vi "G2CPU Treshold Detection.vi"(4 "Auto Release Treshold Parameters (Enabled)":T3={"Auto Release Treshold (Enabled)"=TRUE, "Auto Release Rising Edge (Enabled)"=TRUE}, 6 "Auto Release Line Profiles (Enabled)":T2={"Auto Release Line Profiles (Enabled)"=TRUE, "Auto Release Keys (Enabled)"=TRUE}, 8 "error in (no error)":errorcluster, 10 "Treshold Parameters":T1, 11 "Line Profiles":T4) -> (0 "error out":errorcluster, 3 "Edge Indexes out":refnum<class "1D Array f32.lvclass">)   [LabVIEW 2020, in "G2CPU Line Profile.lvlib"]
doc: "Find the location of the first treshold transition in each provided line profile.\nThe treshold parameters are executed on a per key basis.\nThe edge indexes put out are the indexes in the line profile where the treshold is found."
uses:
  G2CPU Line Profile.lvlib
  <vilib>/Natan Biesmans/G2CPU GPU and CPU HPC Toolkit/G2CPU Libraries/Arrays/1DArray/f32/1D Array f32.lvclass
  C:/Program Files/National Instruments/LabVIEW 2025/vi.lib/Natan Biesmans/G2CPU GPU and CPU HPC Toolkit/G2CPU Libraries/Arrays/Array/Array Prototype.lvclass
  <vilib>/Natan Biesmans/G2CPU GPU and CPU HPC Toolkit/G2CPU Libraries/Arrays/2DArray/f32/2D Array f32.lvclass
  <vilib>/Natan Biesmans/G2CPU GPU and CPU HPC Toolkit/G2CPU Libraries/Arrays/2DArray/u32/2D Array u32.lvclass
  <vilib>/Natan Biesmans/G2CPU GPU and CPU HPC Toolkit/G2CPU Libraries/Arrays/1DArray/binary/1D Array binary.lvclass
  <vilib>/Natan Biesmans/G2CPU GPU and CPU HPC Toolkit/G2CPU Libraries/Arrays/1DArray/s32/1D Array s32.lvclass
  <vilib>/Natan Biesmans/G2CPU GPU and CPU HPC Toolkit/G2CPU Libraries/Arrays/Array/Array Prototype.lvclass/Array Prototype.ctl
  d899a25e-58d2-4af9-a8d1-4a182ea10fc8.vi
  a0a0600d-4521-4ad1-868a-d08d3e0fc7ce.vi
  ee5f6664-b0a7-4185-b73b-108c1a354337.vi
  dc3a3043-0922-4d92-8bdc-4d35e29345f6.vi
  c8160532-a8a2-4c2d-9996-77c21ebed38b.vi
  7a05fecc-ed5d-4a87-a0b2-d0c328027071.vi
  <vilib>/Natan Biesmans/G2CPU GPU and CPU HPC Toolkit/G2CPU Libraries/Arrays/Array/G2CPU Get Array Pointer.vi
  d899a25e-58d2-4af9-a8d1-4a182ea10fc8.vi/2e03f477-51b7-4ba0-bb4f-4f838f6557e6.vi
  d899a25e-58d2-4af9-a8d1-4a182ea10fc8.vi/125d45d4-836b-469d-8a4a-6adb452f866d.vi
  d899a25e-58d2-4af9-a8d1-4a182ea10fc8.vi/8038e9ed-2e71-4568-91ba-0d873494c5ed.vi
  a0a0600d-4521-4ad1-868a-d08d3e0fc7ce.vi/2e03f477-51b7-4ba0-bb4f-4f838f6557e6.vi
  a0a0600d-4521-4ad1-868a-d08d3e0fc7ce.vi/125d45d4-836b-469d-8a4a-6adb452f866d.vi
  a0a0600d-4521-4ad1-868a-d08d3e0fc7ce.vi/8038e9ed-2e71-4568-91ba-0d873494c5ed.vi
  ee5f6664-b0a7-4185-b73b-108c1a354337.vi/cf27cc0d-1fb9-4e2f-ac40-7e8a0db6b27f.vi
  ee5f6664-b0a7-4185-b73b-108c1a354337.vi/1874d702-7e82-49f0-9e52-8a9dc00bddc1.vi
  ee5f6664-b0a7-4185-b73b-108c1a354337.vi/d603c635-5557-46f9-9702-9944444483a4.vi
  dc3a3043-0922-4d92-8bdc-4d35e29345f6.vi/a7ec311c-7cd8-4650-9526-d70ff0a769d1.vi
  c8160532-a8a2-4c2d-9996-77c21ebed38b.vi/5793b77b-c002-4ebf-9075-685617c95341.vi
  c8160532-a8a2-4c2d-9996-77c21ebed38b.vi/2ed3ef86-c00d-4d71-b84c-20267a6dfcf9.vi
  7a05fecc-ed5d-4a87-a0b2-d0c328027071.vi/d8e2d9cc-c923-495e-b121-b6b84788c73f.vi
  7a05fecc-ed5d-4a87-a0b2-d0c328027071.vi/345e91f0-9a5e-4de4-af9c-133346717e4a.vi
  d899a25e-58d2-4af9-a8d1-4a182ea10fc8.vi/2e03f477-51b7-4ba0-bb4f-4f838f6557e6.vi/d8e2d9cc-c923-495e-b121-b6b84788c73f.vi
  d899a25e-58d2-4af9-a8d1-4a182ea10fc8.vi/2e03f477-51b7-4ba0-bb4f-4f838f6557e6.vi/345e91f0-9a5e-4de4-af9c-133346717e4a.vi
  a0a0600d-4521-4ad1-868a-d08d3e0fc7ce.vi/2e03f477-51b7-4ba0-bb4f-4f838f6557e6.vi/d8e2d9cc-c923-495e-b121-b6b84788c73f.vi
  a0a0600d-4521-4ad1-868a-d08d3e0fc7ce.vi/2e03f477-51b7-4ba0-bb4f-4f838f6557e6.vi/345e91f0-9a5e-4de4-af9c-133346717e4a.vi
  ee5f6664-b0a7-4185-b73b-108c1a354337.vi/cf27cc0d-1fb9-4e2f-ac40-7e8a0db6b27f.vi/3e802c67-fb96-46a3-ae13-4994a8508b4f.vi
  ee5f6664-b0a7-4185-b73b-108c1a354337.vi/cf27cc0d-1fb9-4e2f-ac40-7e8a0db6b27f.vi/5a50fc67-79e7-4972-80c2-92243cd53dd4.vi
  ee5f6664-b0a7-4185-b73b-108c1a354337.vi/cf27cc0d-1fb9-4e2f-ac40-7e8a0db6b27f.vi/4b7910ad-0c4a-46e4-b1b3-c9721aeaa91e.vi
  ee5f6664-b0a7-4185-b73b-108c1a354337.vi/1874d702-7e82-49f0-9e52-8a9dc00bddc1.vi/77c7badc-ed81-4514-99c1-20d37f4e5ecc.vi
  ee5f6664-b0a7-4185-b73b-108c1a354337.vi/1874d702-7e82-49f0-9e52-8a9dc00bddc1.vi/eb76fa01-6782-47b4-b34f-9eb474c9cc78.vi
  <vilib>/Natan Biesmans/G2CPU GPU and CPU HPC Toolkit/ArrayFire Driver/VIs/Run as Multi Device.vi
  ee5f6664-b0a7-4185-b73b-108c1a354337.vi/d603c635-5557-46f9-9702-9944444483a4.vi/730f6c57-5c0b-4ee9-b61e-75067b25222b.vi
  ee5f6664-b0a7-4185-b73b-108c1a354337.vi/d603c635-5557-46f9-9702-9944444483a4.vi/096b8799-7810-404e-baca-ba9279cec4bd.vi
  ee5f6664-b0a7-4185-b73b-108c1a354337.vi/d603c635-5557-46f9-9702-9944444483a4.vi/0f1a5a47-bcc5-4796-ac31-8dfcfbc0d7d1.vi
  ee5f6664-b0a7-4185-b73b-108c1a354337.vi/d603c635-5557-46f9-9702-9944444483a4.vi/89f12e17-3330-4b72-ad8f-8dd636660732.vi
  c8160532-a8a2-4c2d-9996-77c21ebed38b.vi/5793b77b-c002-4ebf-9075-685617c95341.vi/3e802c67-fb96-46a3-ae13-4994a8508b4f.vi
  c8160532-a8a2-4c2d-9996-77c21ebed38b.vi/5793b77b-c002-4ebf-9075-685617c95341.vi/5a50fc67-79e7-4972-80c2-92243cd53dd4.vi
  c8160532-a8a2-4c2d-9996-77c21ebed38b.vi/5793b77b-c002-4ebf-9075-685617c95341.vi/4b7910ad-0c4a-46e4-b1b3-c9721aeaa91e.vi
  c8160532-a8a2-4c2d-9996-77c21ebed38b.vi/2ed3ef86-c00d-4d71-b84c-20267a6dfcf9.vi/730f6c57-5c0b-4ee9-b61e-75067b25222b.vi
  c8160532-a8a2-4c2d-9996-77c21ebed38b.vi/2ed3ef86-c00d-4d71-b84c-20267a6dfcf9.vi/096b8799-7810-404e-baca-ba9279cec4bd.vi
  c8160532-a8a2-4c2d-9996-77c21ebed38b.vi/2ed3ef86-c00d-4d71-b84c-20267a6dfcf9.vi/0f1a5a47-bcc5-4796-ac31-8dfcfbc0d7d1.vi
  c8160532-a8a2-4c2d-9996-77c21ebed38b.vi/2ed3ef86-c00d-4d71-b84c-20267a6dfcf9.vi/89f12e17-3330-4b72-ad8f-8dd636660732.vi
  ee5f6664-b0a7-4185-b73b-108c1a354337.vi/cf27cc0d-1fb9-4e2f-ac40-7e8a0db6b27f.vi/5a50fc67-79e7-4972-80c2-92243cd53dd4.vi/1b7cf390-2ae0-48f3-9bce-03c57eed6ee8.vi
  ee5f6664-b0a7-4185-b73b-108c1a354337.vi/d603c635-5557-46f9-9702-9944444483a4.vi/730f6c57-5c0b-4ee9-b61e-75067b25222b.vi/0070e0fe-4ad7-4a3e-8965-d64becb7e5f0.vi
  c8160532-a8a2-4c2d-9996-77c21ebed38b.vi/5793b77b-c002-4ebf-9075-685617c95341.vi/5a50fc67-79e7-4972-80c2-92243cd53dd4.vi/1b7cf390-2ae0-48f3-9bce-03c57eed6ee8.vi
  <vilib>/Natan Biesmans/G2CPU GPU and CPU HPC Toolkit/G2CPU Libraries/Arrays/1DArray/u32/1D Array u32.lvclass
  <vilib>/Natan Biesmans/G2CPU GPU and CPU HPC Toolkit/G2CPU Libraries/Arrays/1DArray/s64/1D Array s64.lvclass
  <vilib>/Natan Biesmans/G2CPU GPU and CPU HPC Toolkit/G2CPU Libraries/Arrays/2DArray/s64/2D Array s64.lvclass
  <vilib>/Natan Biesmans/G2CPU GPU and CPU HPC Toolkit/G2CPU Libraries/Arrays/2DArray/binary/2D Array binary.lvclass
  <vilib>/Natan Biesmans/G2CPU GPU and CPU HPC Toolkit/ArrayFire Driver/VIs/cast.vi
  <vilib>/Natan Biesmans/G2CPU GPU and CPU HPC Toolkit/G2CPU Libraries/Arrays/Array/G2CPU Set Array Pointer.vi
  <vilib>/Natan Biesmans/G2CPU GPU and CPU HPC Toolkit/ArrayFire Driver/VIs/lookup.vi
  <vilib>/Natan Biesmans/G2CPU GPU and CPU HPC Toolkit/ArrayFire Driver/VIs/iszero.vi
  <vilib>/Natan Biesmans/G2CPU GPU and CPU HPC Toolkit/ArrayFire Driver/VIs/sub.vi
  <vilib>/Natan Biesmans/G2CPU GPU and CPU HPC Toolkit/ArrayFire Driver/VIs/release array.vi
  <vilib>/Natan Biesmans/G2CPU GPU and CPU HPC Toolkit/ArrayFire Driver/subvi/Error Converter (ErrCode or Status).vi
  <vilib>/Natan Biesmans/G2CPU GPU and CPU HPC Toolkit/ArrayFire Driver/VIs/add.vi
  <vilib>/Natan Biesmans/G2CPU GPU and CPU HPC Toolkit/ArrayFire Driver/VIs/accum.vi
  <vilib>/Natan Biesmans/G2CPU GPU and CPU HPC Toolkit/G2CPU Libraries/Arrays/SubVI/RemoveReducedDimensionForReorder.vi
  <vilib>/Natan Biesmans/G2CPU GPU and CPU HPC Toolkit/ArrayFire Driver/VIs/reorder.vi
  <vilib>/Natan Biesmans/G2CPU GPU and CPU HPC Toolkit/G2CPU Libraries/Arrays/SubVI/is 2D.vi
  <vilib>/Natan Biesmans/G2CPU GPU and CPU HPC Toolkit/ArrayFire Driver/VIs/where.vi
  <vilib>/Natan Biesmans/G2CPU GPU and CPU HPC Toolkit/G2CPU Libraries/Arrays/SubVI/is 1D.vi
  <vilib>/Natan Biesmans/G2CPU GPU and CPU HPC Toolkit/G2CPU Libraries/Arrays/Array/Array Prototype.lvclass
  <vilib>/Natan Biesmans/G2CPU GPU and CPU HPC Toolkit/G2CPU Libraries/Arrays/DataTypes/I32/s32.lvclass
  <vilib>/Natan Biesmans/G2CPU GPU and CPU HPC Toolkit/G2CPU Libraries/Arrays/1DArray/1D Array Prototype.lvclass
  <vilib>/Natan Biesmans/G2CPU GPU and CPU HPC Toolkit/G2CPU Libraries/Arrays/2DArray/2D Array Prototype.lvclass
  <vilib>/Natan Biesmans/G2CPU GPU and CPU HPC Toolkit/G2CPU Libraries/Arrays/DataTypes/I64/s64.lvclass
  <vilib>/Natan Biesmans/G2CPU GPU and CPU HPC Toolkit/G2CPU Libraries/Arrays/DataTypes/f32/f32.lvclass
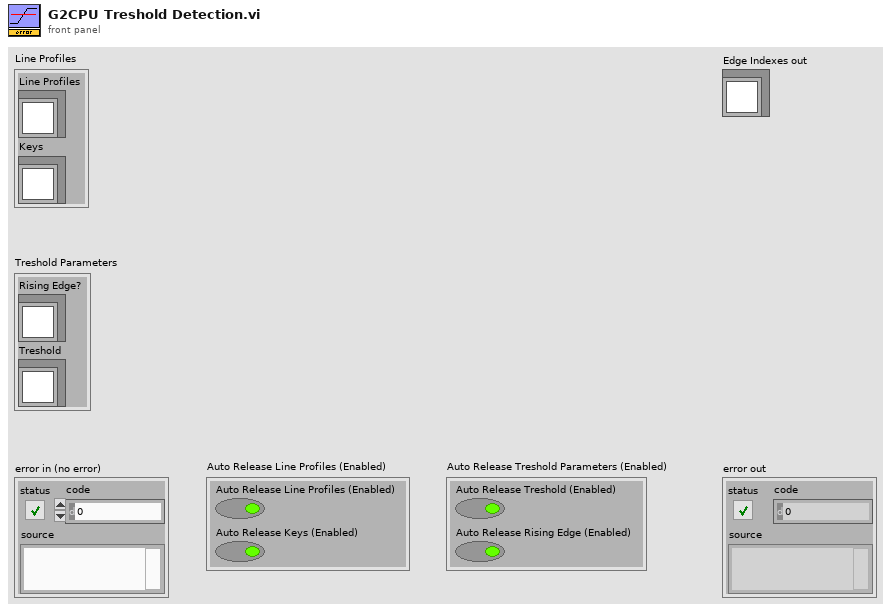
[diagram p1: front panel]
types:
  T1 = cluster{"Rising Edge?":refnum<class "1D Array binary.lvclass">, "Treshold":refnum<class "1D Array s32.lvclass">}
  T2 = cluster{"Auto Release Line Profiles (Enabled)":bool, "Auto Release Keys (Enabled)":bool}
  T3 = cluster{"Auto Release Treshold (Enabled)":bool, "Auto Release Rising Edge (Enabled)":bool}
  T4 = cluster{"Line Profiles":refnum<class "2D Array f32.lvclass">, "Keys":refnum<class "2D Array u32.lvclass">}
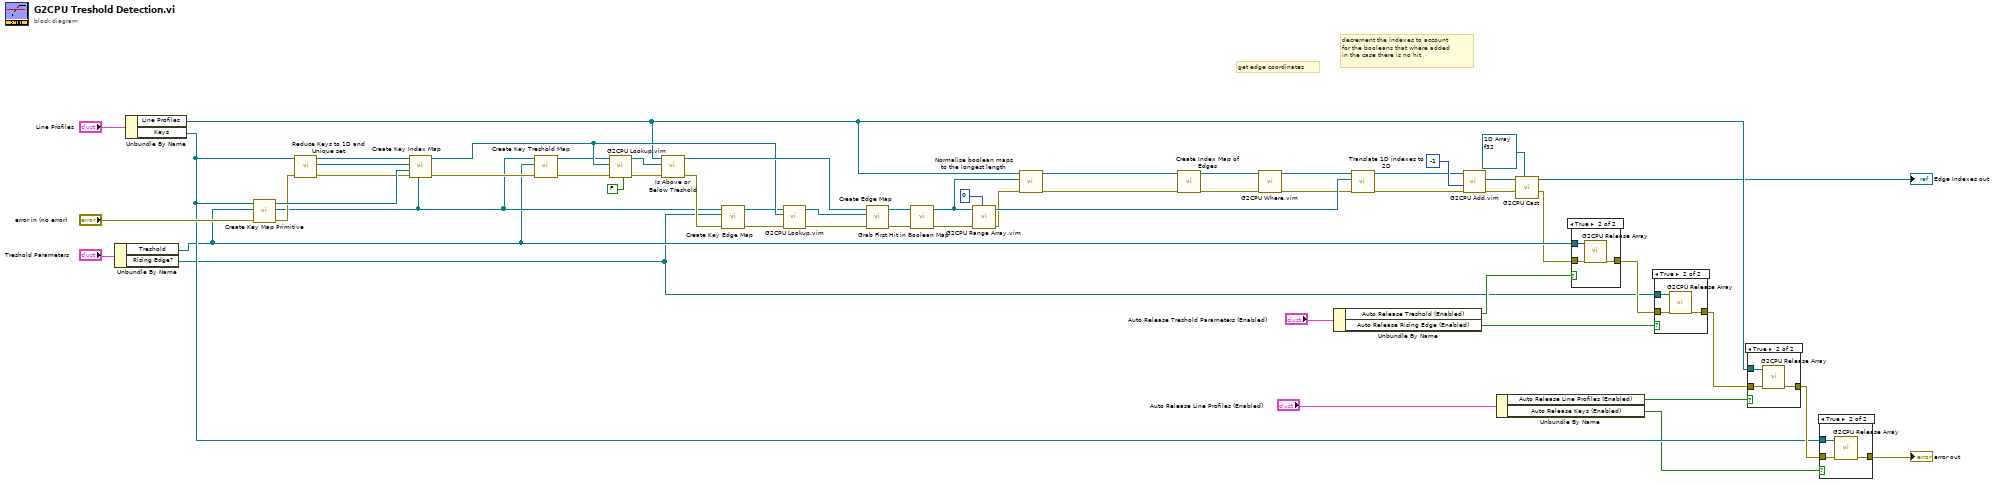
[diagram p0: block diagram]
diagram:
  # "decrement the indexes to account\nfor the booleans that where added\nin the case there is no hit"
  # "get edge coordinates"
  n1 = Unbundle By Name("Treshold Parameters") -> ("Treshold"=w5:refnum<class "1D Array s32.lvclass">, "Rising Edge?"=w4:refnum<class "1D Array binary.lvclass">)
  n2 = Unbundle By Name("Line Profiles") -> ("Line Profiles"=w3:refnum<class "2D Array f32.lvclass">, "Keys"=w13:refnum<class "2D Array u32.lvclass">)
  n3 = call "Create Key Map Primitive.vi"("error in (no error)"="error in (no error)", "Tresholds"=w5, "Keys"=w13) -> ("error out"=w24:errorcluster, "Transposed Key MapPrimitive"=w21:refnum<class "2D Array u32.lvclass">, "Key Map Primitive"=w27:refnum<class "2D Array u32.lvclass">)  [unwired: 6 in]
  n4 = call "Reduce Keys to 1D and Unique set.vi"("error in (no error)"=w24, "Keys"=w13) -> ("error out"=w25:errorcluster, "Reduced Keys"=w23:refnum<class "1D Array u32.lvclass">, "Unique Keys"=w22:refnum<class "1D Array u32.lvclass">)  [unwired: 7 in]
  n5 = call "Create Key Index Map.vi"("Key Map Transposed Primitive"=w21, "error in (no error)"=w25, "Key Map Primitive"=w27, "Reduced Keys for Each line Profile"=w23, "Unique Keys"=w22) -> ("error out"=w26:errorcluster, "Key Line Profile Indexes"=w36:refnum<class "1D Array u32.lvclass">)  [unwired: 5 in]
  n6 = call "Create Key Treshold Map.vi"("error in (no error)"=w26, "Tresholds"=w5, "Key Map Primitive"=w21) -> ("error out"=w37:errorcluster, "Key Treshold Map"=w35:refnum<class "1D Array u32.lvclass">)  [unwired: 7 in]
  n7 = call "G2CPU Lookup.vim"("Auto Release Indices (Enabled)"=FALSE, "error in (no error)"=w37, "Indices (1D)"=w36, "Array In"=w35) -> ("error out"=w34:errorcluster, "Indexed Array"=w33:refnum<class "1D Array u32.lvclass">)  [unwired: 6 in]
  n8 = call "Is Above or Below Treshold.vi"("error in (no error)"=w34, "Keyed Tresholds"=w33, "Line Profiles"=w3) -> ("error out"=w29:errorcluster, "Is Below Treshold?"=w44:refnum<class "2D Array binary.lvclass">)  [unwired: 7 in]
  n9 = call "Create Key Edge Map.vi"("error in (no error)"=w29, "Rising Edge?"=w4, "Key Map Primitive"=w21) -> ("error out"=w32:errorcluster, "Key Edge Map"=w31:refnum<class "1D Array s64.lvclass">)  [unwired: 7 in]
  n10 = call "G2CPU Lookup.vim"("error in (no error)"=w32, "Indices (1D)"=w36, "Array In"=w31) -> ("error out"=w28:errorcluster, "Indexed Array"=w30:refnum<class "1D Array s64.lvclass">)  [unwired: 7 in]
  n11 = call "Create Edge Map.vi"("error in (no error)"=w28, "Keyed Edge to Detect"=w30, "Is Value Below Treshold?"=w44) -> ("error out"=w46:errorcluster, "Edge Map"=w45:refnum<class "2D Array binary.lvclass">)  [unwired: 7 in]
  n12 = call "Grab First Hit in Boolean Map.vi"("error in (no error)"=w46, "Boolean Index Map"=w45) -> ("error out"=w41:errorcluster, "Backfilled Boolean Index Map"=w39:refnum<class "2D Array binary.lvclass">)  [unwired: 8 in]
  n13 = call "G2CPU Range Array.vim"("Datatype"=i64 0, "Error in"=w41, "Size"=w39) -> ("error out"=w40:errorcluster, "Array out"=w50:refnum<class "2D Array s64.lvclass">)  [unwired: 7 in]
  n14 = call "Normalise boolean maps to the longest length.vi"("error in (no error)"=w40, "Boolean Index map"=w39, "Line Profiles"=w3) -> ("error out"=w57:errorcluster, "Normalised Boolean Index Map"=w56:refnum<class "2D Array binary.lvclass">)  [unwired: 7 in]
  n15 = call "Create Index Map of Edges.vi"("error in (no error)"=w57, "2D Array binary in"=w56) -> ("error out"=w55:errorcluster, "2D Array binary out"=w54:refnum<class "2D Array binary.lvclass">)  [unwired: 8 in]
  n16 = call "G2CPU Where.vim"("error in (no error)"=w55, "Array in"=w54) -> ("error out"=w48:errorcluster, "Non Zero Indices"=w47:refnum<class "1D Array u32.lvclass">)  [unwired: 8 in]
  n17 = Unbundle By Name("Auto Release Treshold Parameters (Enabled)") -> ("Auto Release Treshold (Enabled)"=w11:bool, "Auto Release Rising Edge (Enabled)"=w10:bool)
  n18 = call "Translate 1D indexes to 2D.vi"("error in (no error)"=w48, "Range Array for Queue size mapping"=w50, "1D Indexes in"=w47) -> ("error out"=w52:errorcluster, "Mapped to 2D indexes out"=w51:refnum<class "1D Array s32.lvclass">)  [unwired: 7 in]
  n19 = call "G2CPU Add.vim"("error in (no error)"=w52, "Array rhs"=-1 ("Datatype Prototype"), "Array lhs"=w51) -> ("error out"=w19:errorcluster, "Array Result"=w20:refnum<class "1D Array s32.lvclass">)  [unwired: 7 in]
  n20 = Unbundle By Name("Auto Release Line Profiles (Enabled)") -> ("Auto Release Line Profiles (Enabled)"=w8:bool, "Auto Release Keys (Enabled)"=w7:bool)
  n21 = call "G2CPU Cast"("Datatype Prototype"=refnum<class "1D Array f32.lvclass"> refnum ("G2CPU Arrays.lvlib:1D Array f32.lvclass"), "error in (no error)"=w19, "Array In"=w20) -> ("error out"=w1:errorcluster, "Array Out"=→"Edge Indexes out":refnum<class "1D Array f32.lvclass">)  [unwired: 7 in]
  n22 = case shown="True" w11 {
    tunnel: w5 -> [_ w61]
    tunnel: w1 -> [w58 w60]
    tunnel: [w58 w59] -> w17
    frame False {
    }
    frame True {
      n23 = call <vilib>:"G2CPU Release Array.vi"("error in (no error)"=w60, "Array in"=w61) -> ("error out"=w59:errorcluster)  [unwired: 9 in]
    }
  }
  n24 = case shown="True" w10 {
    tunnel: w4 -> [_ w65]
    tunnel: w17 -> [w62 w64]
    tunnel: [w62 w63] -> w16
    frame False {
    }
    frame True {
      n25 = call <vilib>:"G2CPU Release Array.vi"("error in (no error)"=w64, "Array in"=w65) -> ("error out"=w63:errorcluster)  [unwired: 9 in]
    }
  }
  n26 = case shown="True" w8 {
    tunnel: w3 -> [_ w69]
    tunnel: w16 -> [w66 w68]
    tunnel: [w66 w67] -> w15
    frame False {
    }
    frame True {
      n27 = call <vilib>:"G2CPU Release Array.vi"("error in (no error)"=w68, "Array in"=w69) -> ("error out"=w67:errorcluster)  [unwired: 9 in]
    }
  }
  n28 = case shown="True" w7 {
    tunnel: w13 -> [_ w73]
    tunnel: w15 -> [w70 w72]
    tunnel: [w70 w71] -> w14
    frame False {
    }
    frame True {
      n29 = call <vilib>:"G2CPU Release Array.vi"("error in (no error)"=w72, "Array in"=w73) -> ("error out"=w71:errorcluster)  [unwired: 9 in]
    }
  }
  "error out" <- w14
